vi "mxwScript_API_XMLTemplateName_AddNewDiagramRef.vi"(8 "error in (no error)":errorcluster, 9 "path":string, 10 "uniqueID":string, 11 "absolutePath":string) -> (0 "error out":errorcluster, 3 "encoded absolutePath":string)   [LabVIEW 2017]
doc: "Use the <B>path</B> to find a diagram on the template after it is dropped, then store a reference to it under <B>uniqueID</B> in the diagram reference array."
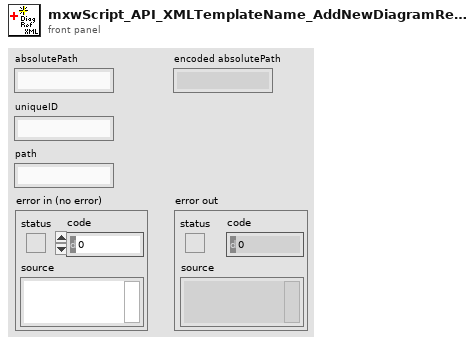
[diagram p1: front panel]
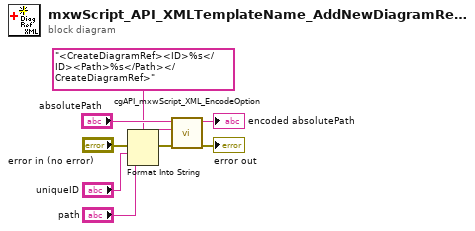
[diagram p0: block diagram]
diagram:
  n1 = Format Into String(format string="<CreateDiagramRef><ID>%s</ID><Path>%s</Path></CreateDiagramRef>" ("control name"), error in="error in (no error)", "uniqueID", "path") -> (resulting string=w4:string, error out=w6:errorcluster)  [unwired: 1 in]
  n2 = call "cgAPI_mxwScript_XML_EncodeOption.vi"("error in (no error)"=w6, "otherXML"=w4, "normalTextString"="absolutePath") -> ("error out"=→"error out":errorcluster, "encodedString"=→"encoded absolutePath":string)  [unwired: 7 out]
